vi "Intake Get and use.vi"(2 "TakeBall":dbl, 3 "Cannon vbus":dbl, 4 "Upper Claw":dbl) -> (0 "Intake Info Out":T1, 1 "InTake Max":bool)   [LabVIEW 2013]
uses:
  Intake Global.vi
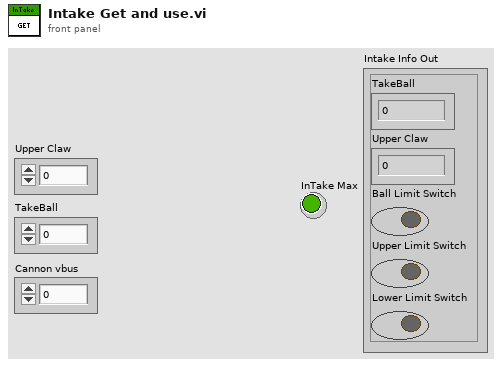
[diagram p1: front panel]
types:
  T1 = cluster{"TakeBall":dbl, "Upper Claw":dbl, "Ball Limit Switch":bool, "Upper Limit Switch":bool, "Lower Limit Switch ":bool}
  T2 = cluster{"TakeBall":dbl, "Upper Claw":dbl, "Ball In Cannon?":bool, "InTake Max":bool, "InTake Min":bool}
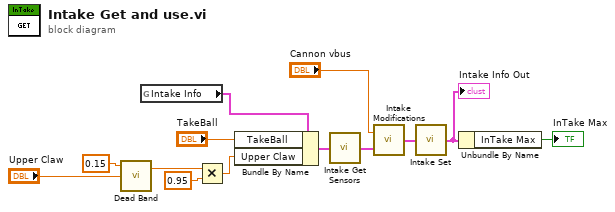
[diagram p0: block diagram]
diagram:
  n1 = call "Dead Band.vi"("Axis 1 In"="Upper Claw", "Dead Band"=0.15) -> ("Axis 1 Out"=w3:dbl)  [unwired: 1 in, 1 out]
  n2 = global read "Intake Global.vi" "Intake Info"() -> (w13:T2)
  n3 = Multiply(x=w3, y=0.95) -> (x*y=w1:dbl)
  n4 = Bundle By Name(cluster=w13, "TakeBall"="TakeBall", "Upper Claw"=w1) -> (w11:T2)
  n5 = call "Intake Get Sensors.vi"("Intake Info In"=w11) -> ("Intake Info In"=w10:T2)
  n6 = call "Intake Modifications.vi"("Intake Info In"=w10, "Cannon vbus"="Cannon vbus") -> ("Intake Info In"=w7:T2)
  n7 = call "Intake Set.vi"("Intake Info In"=w7) -> ("Intake Info In"=w6:T2)
  "Intake Info Out" <- w6
  n8 = Unbundle By Name(w6) -> ("InTake Max"=→"InTake Max":bool)
